vi "U32 to DBL.vi"(2 "U32":u32) -> (6 "DBL":dbl)   [LabVIEW 2019, in "Modbus.lvclass"]
uses:
  Modbus.lvclass
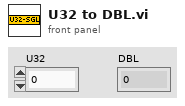
[diagram p1: front panel]
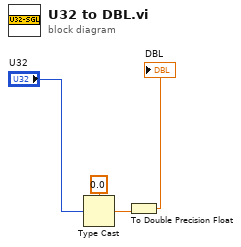
[diagram p0: block diagram]
diagram:
  n1 = Type Cast(type=sgl 0.0 ("double precision float"), x="U32") -> (*(type *) &x=w4:sgl)
  n2 = To Double Precision Float(number=w4) -> (double precision float=→"DBL":dbl)
